vi "Flush Client Handles.vi"(8 "error in (no error)":errorcluster, 11 "REST Client in":refnum<class "REST Client.lvclass">) -> (0 "error out":errorcluster, 3 "REST Client out":refnum<class "REST Client.lvclass">)   [LabVIEW 2020, in "REST Client.lvlib" / "REST Client.lvclass"]
doc: "Destroy REST client reference."
uses:
  REST Client.lvclass
  REST Client.lvclass/REST Client.ctl
  <vilib>/VIPM Community/HTTP Client Plugin - Base/Classes/Abstract HTTP Client/Abstract HTTP Client.lvclass
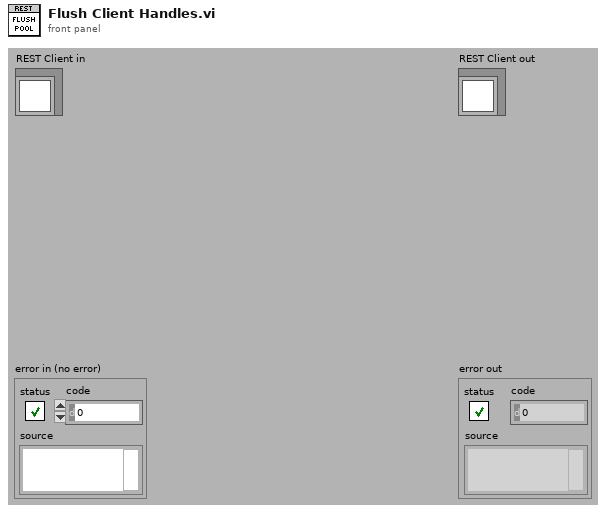
[diagram p1: front panel]
types:
  T1 = typedef "REST Client.lvlib/REST Client.lvclass/HTTP Header.ctl" = cluster{"header":T2, "value":string}
  T2 = typedef "lib_NI_Advanced HTTP Client.lvlib/Session.lvclass/Header--Combo Box.ctl" = string
  T3 = cluster{"HTTP Client Abstract.lvlib:Abstract HTTP Client.lvclass":refnum<class "Abstract HTTP Client.lvclass">, "Default Headers ([JSON])":T1[]}[]
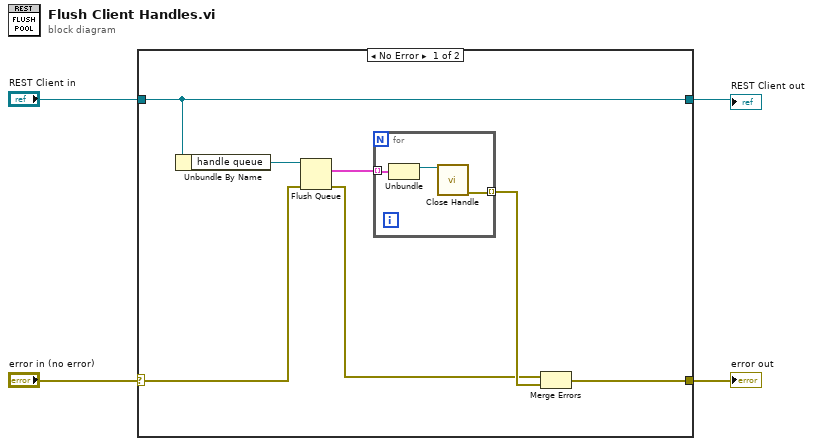
[diagram p0: block diagram]
diagram:
  n1 = case shown="No Error" "error in (no error)" {
    selector: "error in (no error)" -> [w6 w15]
    tunnel: "REST Client in" -> [w7 w16]
    tunnel: [w9 w15] -> w3
    tunnel: [w7 w16] -> w1
    frame No Error {
      n2 = Unbundle By Name(w7) -> ("handle queue"=w11:refnum<queue>)
      n3 = Flush Queue(queue=w11, error in (no error)=w6) -> (remaining elements=w10:T3, error out=w5:errorcluster)  [unwired: 1 out]
      n4 = for {
        tunnel: w10 -> [w14] mode=indexing
        tunnel: [w12] -> w8 mode=indexing
        n5 = Unbundle(w14) -> ("HTTP Client Abstract.lvlib:Abstract HTTP Client.lvclass"=w13:refnum<class "Abstract HTTP Client.lvclass">)  [unwired: 1 out]
        n6 = call-dynamic "Close Handle.vi"("HTTP Client Abstract in"=w13) -> ("error out"=w12:errorcluster)  [unwired: 9 in, 1 out]
      }
      n7 = Merge Errors(w5, w8) -> (w9:errorcluster)
    }
    frame Error {
    }
  }
  "error out" <- w3
  "REST Client out" <- w1
